vi "ShrimpCam_TakeImage.vi"(0 "Ref (cam in)":refnum<k24>, 1 "Error In":errorcluster) -> (2 "Ref (cam out)":refnum<k24>, 3 "Image":picture, 4 "Error Out":errorcluster)   [LabVIEW 2018]
uses:
  C:/Users/user/Desktop/Thorcam/uc480DotNet.dll
  Thorcam/uc480DotNet.dll
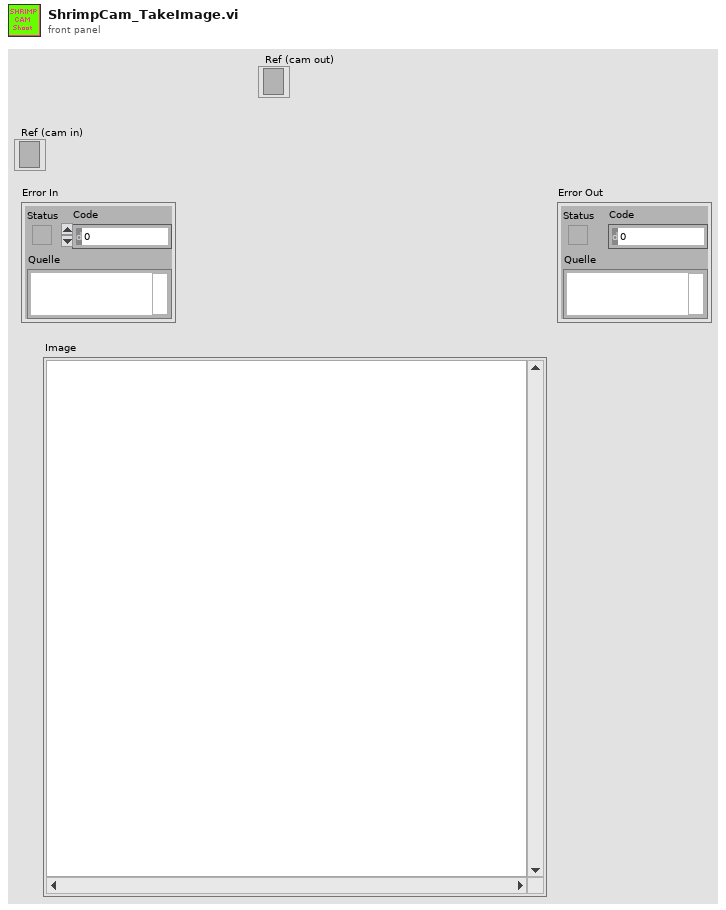
[diagram p1: front panel]
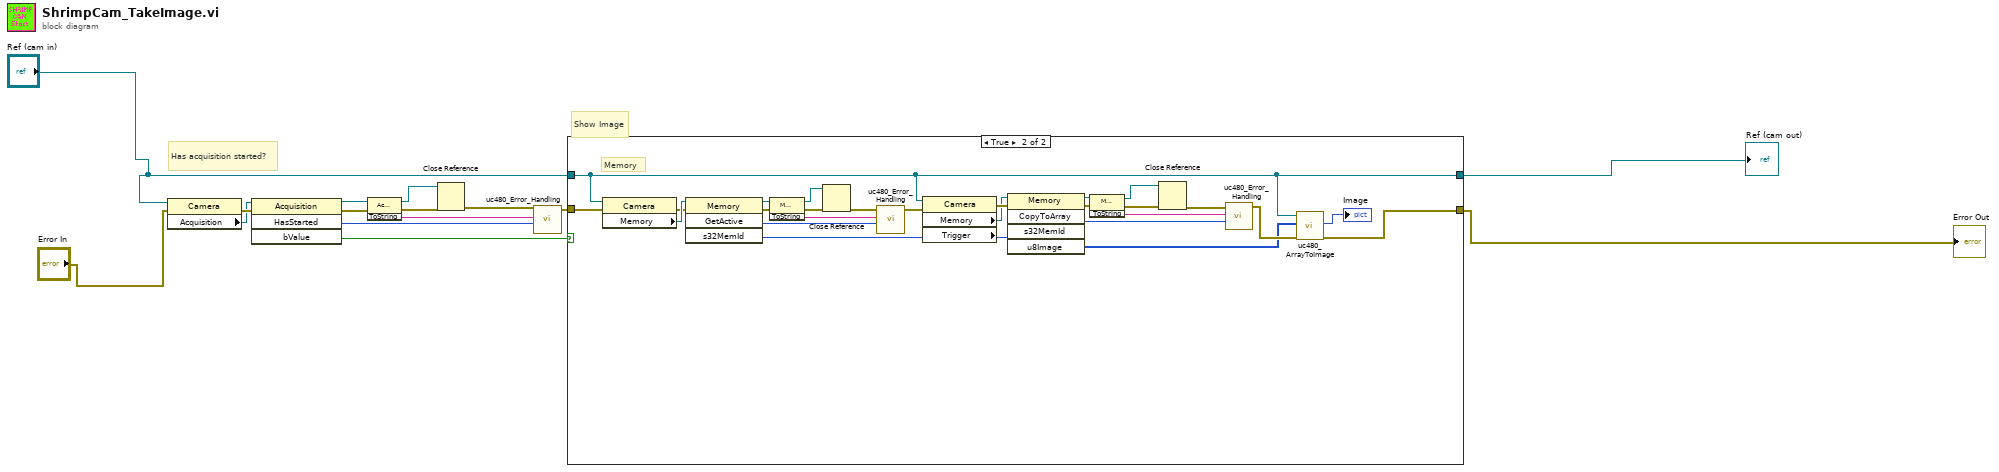
[diagram p0: block diagram]
diagram:
  # "Has acquisition started?"
  # "Show Image"
  n1 = property class="Camera"(reference="Ref (cam in)", error in="Error In") -> (error out=w15:errorcluster, "Acquisition"=w14:refnum<k24>)  [unwired: 1 out]
  n2 = invoke class="Acquisition" method="HasStarted"(reference=w14, error in=w15) -> (reference out=w11:refnum<k24>, error out=w10:errorcluster, "HasStarted"=w9:i32, "bValue"=w13:bool)  [unwired: 2 in]
  n3 = invoke class="Acquisition" method="ToString"(reference=w11, error in=w10) -> (reference out=w5:refnum<k24>, error out=w7:errorcluster, "ToString"=w12:string)  [unwired: 1 in]
  n4 = Close Reference(reference=w5, error in (no error)=w7) -> (error out=w6:errorcluster)
  n5 = call "uc480_Error_Handling.vi"("Error Code"=w9, "Error String"=w12, "Error In"=w6) -> ("Error Out"=w8:errorcluster)  [unwired: 8 in]
  n6 = case shown="True" w13 {
    tunnel: [w17 w29] -> w2
    tunnel: w8 -> [w17 w18]
    tunnel: "Ref (cam in)" -> [w16 w27]
    tunnel: [w16 w27] -> w1
    frame False {
    }
    frame True {
      # "Memory"
      n7 = property class="Camera"(reference=w27, error in=w18) -> (error out=w31:errorcluster, "Memory"=w32:refnum<k24>)  [unwired: 1 out]
      n8 = invoke class="Memory" method="GetActive"(reference=w32, error in=w31) -> (reference out=w37:refnum<k24>, error out=w36:errorcluster, "GetActive"=w38:i32, "s32MemId"=w30:i32)  [unwired: 2 in]
      n9 = invoke class="Memory" method="ToString"(reference=w37, error in=w36) -> (reference out=w23:refnum<k24>, error out=w25:errorcluster, "ToString"=w35:string)  [unwired: 1 in]
      n10 = Close Reference(reference=w23, error in (no error)=w25) -> (error out=w24:errorcluster)
      n11 = call "uc480_Error_Handling.vi"("Error Code"=w38, "Error String"=w35, "Error In"=w24) -> ("Error Out"=w39:errorcluster)  [unwired: 8 in]
      n12 = property class="Camera" props=["Memory", "Trigger"](reference=w27, error in=w39) -> (error out=w34:errorcluster, "Memory"=w33:refnum<k24>)  [unwired: 2 out]
      n13 = invoke class="Memory" method="CopyToArray"(reference=w33, error in=w34, "s32MemId"=w30) -> (reference out=w41:refnum<k24>, error out=w42:errorcluster, "CopyToArray"=w43:i32, "u8Image"=w26:u8[])  [unwired: 2 in, 1 out]
      n14 = invoke class="Memory" method="ToString"(reference=w41, error in=w42) -> (reference out=w20:refnum<k24>, error out=w22:errorcluster, "ToString"=w40:string)  [unwired: 1 in]
      n15 = Close Reference(reference=w20, error in (no error)=w22) -> (error out=w21:errorcluster)
      n16 = call "uc480_Error_Handling.vi"("Error Code"=w43, "Error String"=w40, "Error In"=w21) -> ("Error Out"=w28:errorcluster)  [unwired: 8 in]
      n17 = call "uc480_ArrayToImage.vi"("Error In"=w28, "InArray"=w26, ".NET (Reference)"=w27) -> ("Error Out"=w29:errorcluster, "Image"=→"Image":picture)  [unwired: 7 in]
    }
  }
  "Error Out" <- w2
  "Ref (cam out)" <- w1
